vi "Write Event Handler.vi"(10 "EventHandler":refnum<class "IEventHandler.lvclass">, 11 "IEventAggregator in":refnum<class "IEventAggregator.lvclass">) -> (3 "IEventAggregator out":refnum<class "IEventAggregator.lvclass">)   [LabVIEW 2019, in "ActorEvents.lvlib" / "IEventAggregator.lvclass"]
uses:
  <vilib>/gpm_packages/@cs/mva-viewable/Source/ActorEvents/IEventAggregator/IEventAggregator.lvclass
  <vilib>/gpm_packages/@cs/mva-viewable/Source/ActorEvents/IEventHandler/IEventHandler.lvclass
  <vilib>/gpm_packages/@cs/mva-viewable/Source/ActorEvents/IEventAggregator/IEventAggregator.lvclass/IEventAggregator.ctl
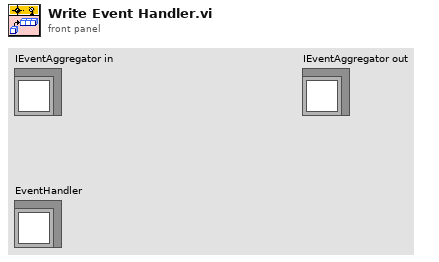
[diagram p1: front panel]
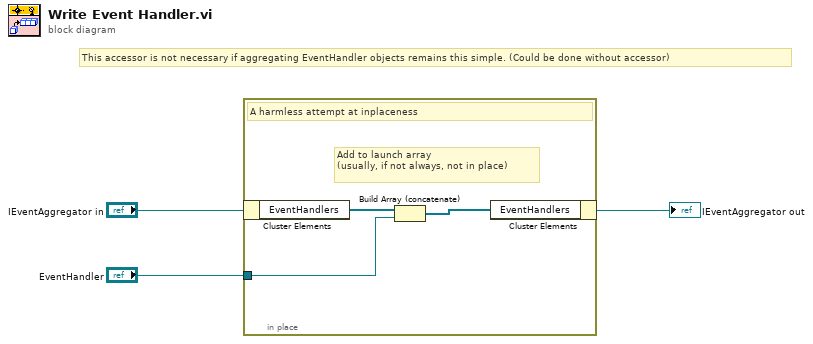
[diagram p0: block diagram]
diagram:
  # "This accessor is not necessary if aggregating EventHandler objects remains this simple. (Could be done without accessor)"
  n1 = in-place {
    in-place-border: "EventHandler" -> [w6]
    # "Add to launch array\n(usually, if not always, not in place)"
    # "A harmless attempt at inplaceness"
    n2 = in-place-cluster #1("IEventAggregator in") -> ("EventHandlers"=w5:refnum<class "IEventHandler.lvclass">[])
    n3 = Build Array (concatenate)(w5, w6) -> (w4:refnum<class "IEventHandler.lvclass">[])
    n4 = in-place-cluster #1("EventHandlers"=w4) -> (→"IEventAggregator out":refnum<class "IEventAggregator.lvclass">)
  }
